vi "零件入库.vi"(8 "error in (no error)":errorcluster caption="错误输入（无错误）", 11 "齿轮 输入":refnum<class "齿轮.lvclass"> caption="DNL_LabVIEW Object in") -> (0 "error out":errorcluster caption="错误输出", 2 "零件入库":string, 3 "齿轮 输出":refnum<class "齿轮.lvclass"> caption="DNL_LabVIEW Object out")   [LabVIEW 2013, in "齿轮.lvclass"]
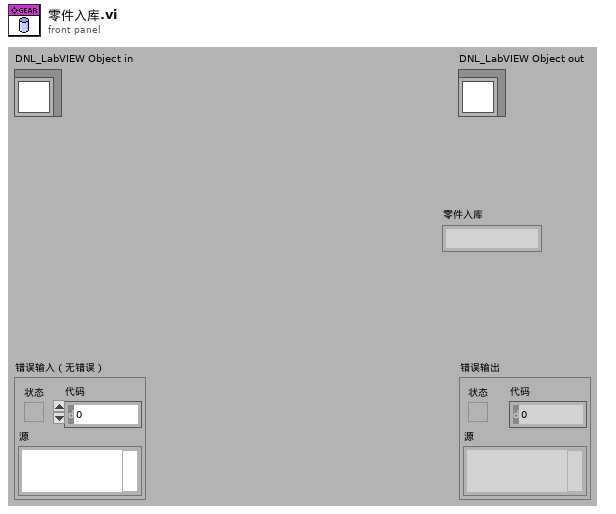
[diagram p1: front panel]
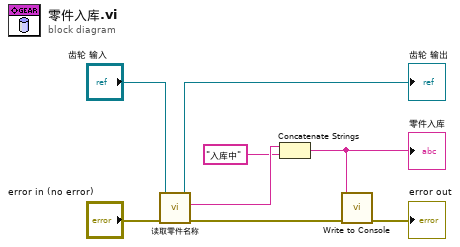
[diagram p0: block diagram]
diagram:
  n1 = call "读取零件名称.vi"("error in (no error)"="error in (no error)", "零件加工（抽象）输入"="齿轮 输入") -> ("error out"=w7:errorcluster, "零件名称"=w3:string, "零件加工（抽象）输出"=→"齿轮 输出":refnum<class "齿轮.lvclass">)  [unwired: 7 in]
  n2 = Concatenate Strings(w3, "入库中" ("字符串")) -> (w1:string)
  "零件入库" <- w1
  n3 = call "Write to Console.vi"("error in (no error)"=w7, "Input"=w1) -> ("error out"=→"error out":errorcluster)  [unwired: 9 in]
